vi "PH_PLH-AccessInformation.calc information.vi"(0 "i ref in":refnum<vi>, 5 "error in":errorcluster) -> (14 "i ref out":refnum<vi>, 16 "Mode":T1(ring), 19 "error out":errorcluster)   [LabVIEW 2014, in "PH_PLH-AccessInformation.lvlib"]
doc: "Calculates the access status out of the information."
uses:
  PH_PLH-AccessInformation.lvlib
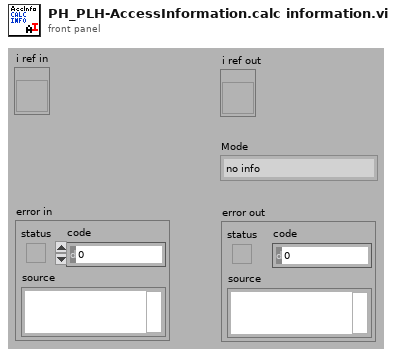
[diagram p1: front panel]
types:
  T1 = enum16{"no info", "free access", "Searchmode", "Shotmode"}
  T2 = typedef "PH_PLH-AccessInformation.lvlib/PH_PLH-AccessInformation.i attribute.ctl" = cluster{"GUI Refs":cluster{"Ref Shotmode":refnum<vi>, "Ref Searchmode":refnum<vi>}, "Shotmode":i32, "Searchmode":i32}
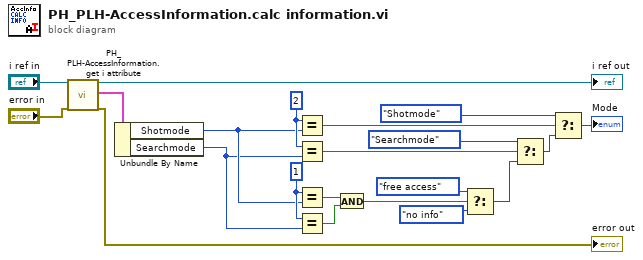
[diagram p0: block diagram]
diagram:
  w10 = 1 ("x")
  w15 = 2 ("x")
  n1 = call "PH_PLH-AccessInformation.get i attribute.vi"("i ref in"="i ref in", "error in (no error)"="error in") -> ("i ref out"=→"i ref out":refnum<vi>, "i attribute"=w19:T2, "error out"=→"error out":errorcluster)  [unwired: 15 in]
  n2 = Unbundle By Name(w19) -> ("Shotmode"=w9:i32, "Searchmode"=w8:i32)
  n3 = Equal?(x=w15, y=w9) -> (x = y?=w12:bool)
  n4 = Equal?(x=w15, y=w8) -> (x = y?=w14:bool)
  n5 = Equal?(x=w10, y=w9) -> (x = y?=w6:bool)
  n6 = Equal?(x=w10, y=w8) -> (x = y?=w5:bool)
  n7 = And(x=w6, y=w5) -> (x .and. y?=w4:bool)
  n8 = Select(t=T1."free access" ("Mode"), s=w4, f=T1."no info" ("Mode")) -> (s? t:f=w3:T1)
  n9 = Select(t=T1."Searchmode" ("Mode"), s=w14, f=w3) -> (s? t:f=w13:T1)
  n10 = Select(t=T1."Shotmode" ("Mode"), s=w12, f=w13) -> (s? t:f=→"Mode":T1)
